vi "Cycle Memory Emulator.vi"(9 "Operation":T1, 10 "Write Data in":u64, 11 "Address":u32) -> (3 "Write Data out":u64)   [LabVIEW 2017, in "FPGA-SRL.lvlib"]
uses:
  FPGA-SRL.lvlib
  user.lib/Utilities/Type Defs/MISC IO Choice Enum.ctl
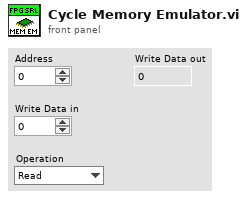
[diagram p1: front panel]
types:
  T1 = typedef "MISC IO Choice Enum.ctl" = enum16{"Read", "Write"}
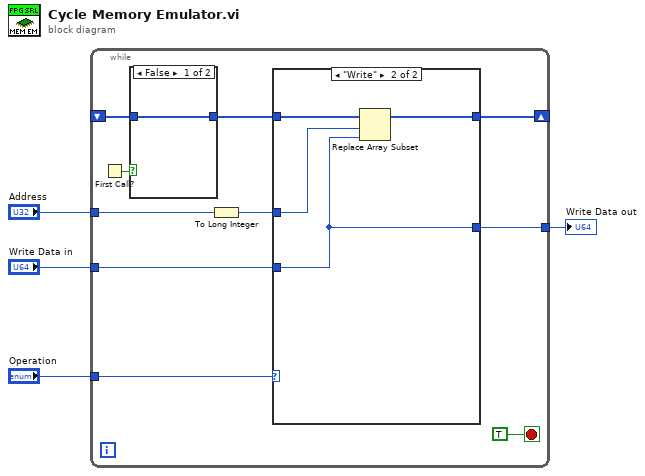
[diagram p0: block diagram]
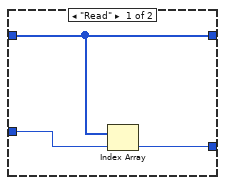
[diagram p2: hidden frame]
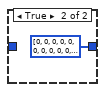
[diagram p3: hidden frame]
diagram:
  n1 = while {
    shift-right: [w9] -> _
    shift-left: _ -> [w13]
    tunnel: "Operation" -> [w10]
    tunnel: "Address" -> [w8]
    tunnel: "Write Data in" -> [w7]
    tunnel: [w5] -> w4
    stop <- TRUE stop-if-true
    n2 = First Call?() -> (First Call?: T/F=w14:bool)
    n3 = case shown="False" w14 {
      tunnel: [w22 u64[] [0, 0, 0, 0, 0, 0, 0, 0, 0, 0, 0, 0, 0, 0, 0, 0, 0, 0, 0, 0, 0, 0, 0, 0, 0, 0, 0, 0, 0, 0, 0, 0, 0, 0, 0, 0, 0, 0, 0, 0, 0, 0, 0, 0, 0, 0, 0, 0, 0, 0, 0, 0, 0, 0, 0, 0, 0, 0, 0, 0, 0, 0, 0, 0, 0, 0, 0, 0, 0, 0, 0, 0, 0, 0, 0, 0, 0, 0, 0, 0, 0, 0, 0, 0, 0, 0, 0, 0, 0, 0, 0, 0, 0, 0, 0, 0]] -> w11
      tunnel: w13 -> [w22 _]
      frame False {
      }
      frame True {
      }
    }
    n4 = To Long Integer(number=w8) -> (32bit integer=w6:i32)
    n5 = case shown="\"Write\"" w10 {
      tunnel: w11 -> [w17 w21]
      tunnel: [w17 w20] -> w9
      tunnel: w6 -> [w16 w19]
      tunnel: w7 -> [_ w18]
      tunnel: [w15 w18] -> w5
      frame "Read" {
        n6 = Index Array(array=w17, index=w16) -> (element=w15:u64)
      }
      frame "Write" {
        n7 = Replace Array Subset(array=w21, new element=w18, index=w19) -> (w20:u64[])
      }
    }
  }
  "Write Data out" <- w4
